vi "请求刷新.vi"(4 "Error Out":errorcluster caption="Error in") -> (0 "title with pic":cluster{"字符串 2":string, "二维图片":picture}[](array[cluster]), 1 "error out":errorcluster, 2 "stories":T1(array[cluster]), 3 "URL":string, 5 "top_stories":cluster{"字符串 2":string, "二维图片":picture}[](array[cluster]))   [LabVIEW 2012]
uses:
  <vilib>/addons/WireFlow/_WF_ProgressBar.llb/MessageTextType.ctl
  <vilib>/addons/WireFlow/_WF_ProgressBar.llb/ProgressBar_WireFlow.lvclass
panel:
  in  "delay (0 ms)":i32=1000
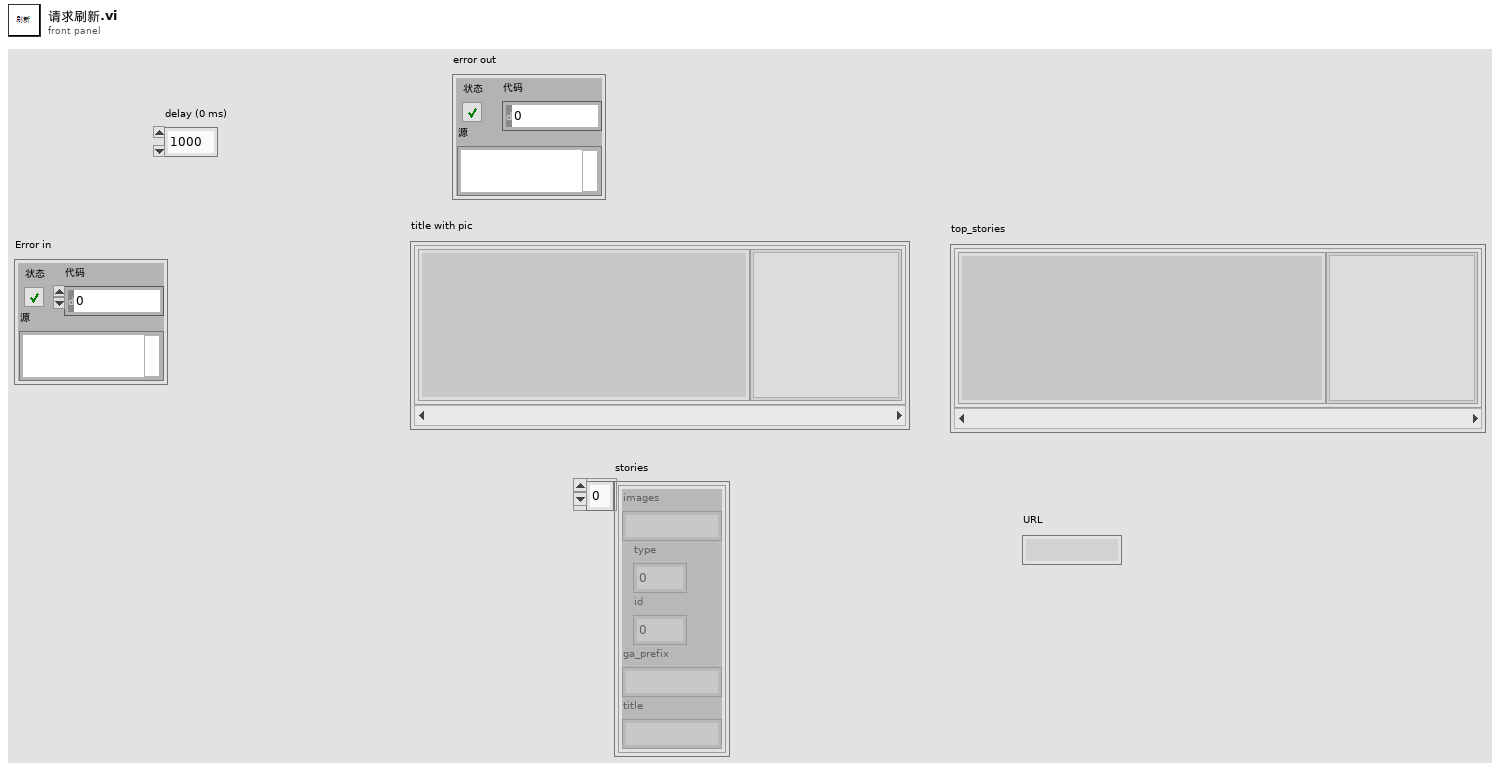
[diagram p1: front panel]
types:
  T1 = cluster{"images":string, "type":i32, "id":i64, "ga_prefix":string, "title":string}[]
  T2 = typedef "ProgressBar_WireFlow.lvclass/MessageTextType.ctl" = enum16{"Title", "General", "Current item"}
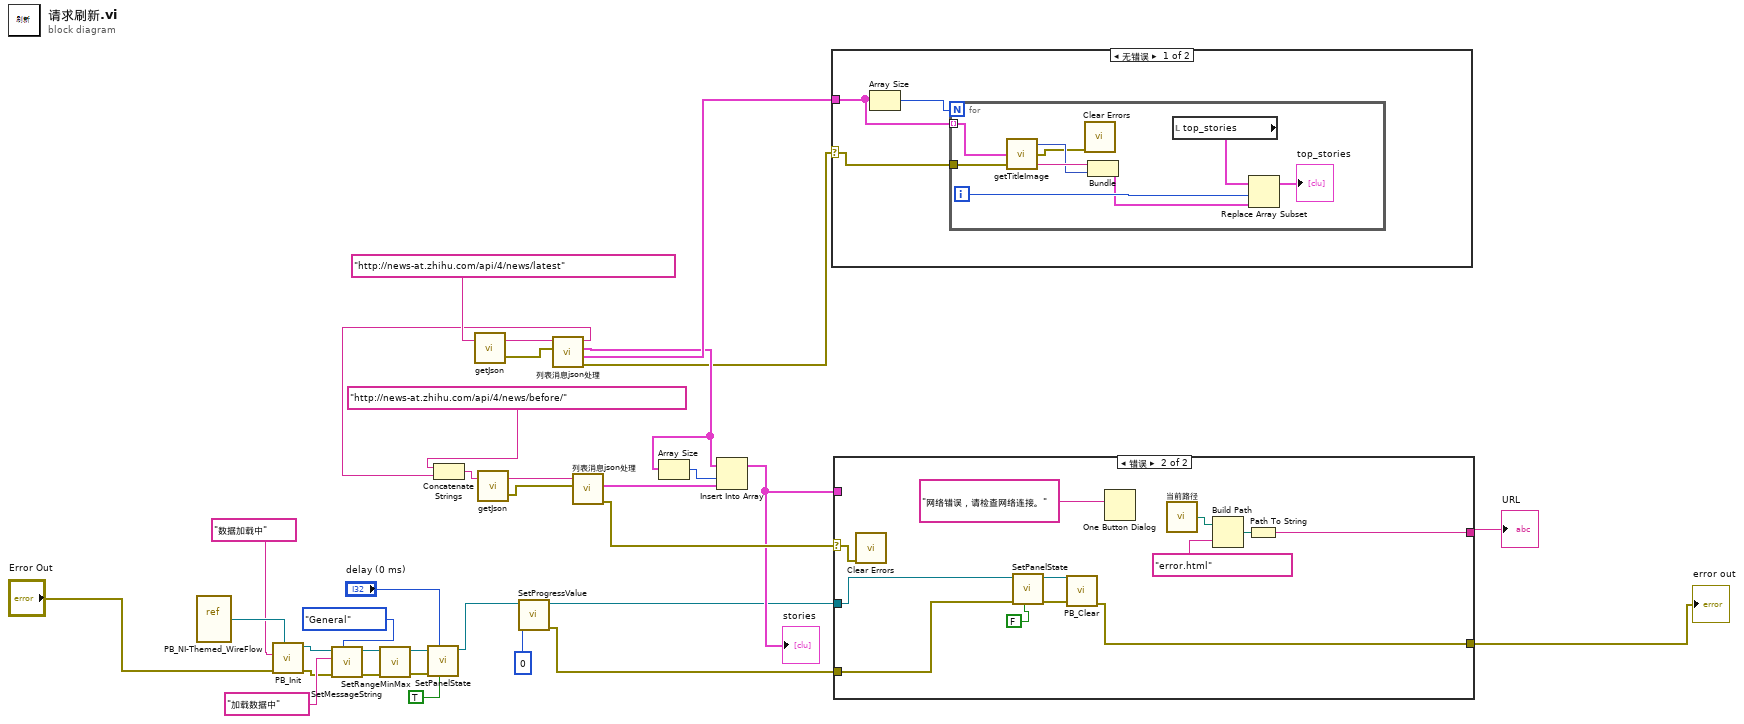
[diagram p0: block diagram]
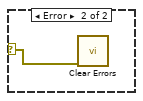
[diagram p2: hidden frame]
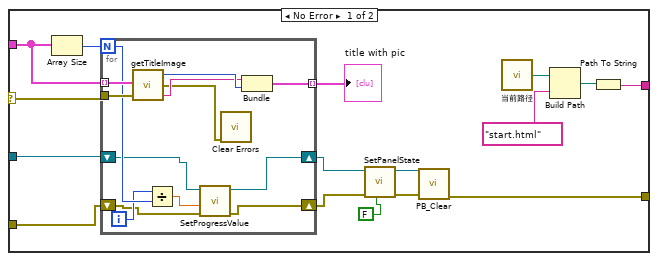
[diagram p3: hidden frame]
diagram:
  n1 = vi-ref "PB_NI-Themed_WireFlow.vi"() -> (w18:refnum<vi>)
  n2 = call <vilib>:"PB_Init.vi"("Progress VI"=w18, "error in (no error)"="Error Out", "title (\"Progress\")"="数据加载中") -> ("error out"=w11:errorcluster, "WF-ProgressBar out"=w16:refnum<class "ProgressBar_WireFlow.lvclass">)  [unwired: 7 in]
  n3 = call-dynamic "SetMessageString.vi"("message field"=MessageTextType."General", "error in (no error)"=w11, "Message"="加载数据中", "WF-ProgressBar in"=w16) -> ("error out"=w12:errorcluster, "WF-ProgressBar out"=w13:refnum<class "ProgressBar_WireFlow.lvclass">)  [unwired: 6 in]
  n4 = call-dynamic "SetRangeMinMax.vi"("error in (no error)"=w12, "WF-ProgressBar in"=w13) -> ("error out"=w9:errorcluster, "WF-ProgressBar out"=w10:refnum<class "ProgressBar_WireFlow.lvclass">)  [unwired: 8 in]
  n5 = call-dynamic "SetPanelState.vi"("State (T = Open)"=TRUE, "delay (0 ms)"="delay (0 ms)", "error in (no error)"=w9, "WF-ProgressBar in"=w10) -> ("WF-ProgressBar out"=w6:refnum<class "ProgressBar_WireFlow.lvclass">)  [unwired: 6 in, 1 out]
  n6 = call "getJson.vi"("URL"="http://news-at.zhihu.com/api/4/news/latest") -> ("error out"=w32:errorcluster, "响应体"=w33:string)  [unwired: 1 in]
  n7 = call-dynamic "SetProgressValue.vi"("Value"=0, "WF-ProgressBar in"=w6) -> ("error out"=w3:errorcluster, "WF-ProgressBar out"=w4:refnum<class "ProgressBar_WireFlow.lvclass">)  [unwired: 7 in, 1 out]
  n8 = call "列表消息json处理.vi"("error in (no error)"=w32, "json input"=w33) -> ("error out"=w22:errorcluster, "top_stories"=w31:T1, "stories"=w24:T1, "date"=w29:string)  [unwired: 2 in]
  n9 = Concatenate Strings("http://news-at.zhihu.com/api/4/news/before/", w29) -> (w30:string)
  n10 = call "getJson.vi"("URL"=w30) -> ("error out"=w26:errorcluster, "响应体"=w27:string)  [unwired: 1 in]
  n11 = call "列表消息json处理.vi"("error in (no error)"=w26, "json input"=w27) -> ("error out"=w23:errorcluster, "stories"=w21:T1)  [unwired: 2 in, 2 out]
  n12 = Array Size(array=w24) -> (size(s)=w25:i32)
  n13 = Insert Into Array(array=w24, index=w25, new element=w21) -> (w19:T1)
  "stories" <- w19
  n14 = case shown="无错误" w22 {
    selector: w22 -> [w35 w47]
    tunnel: w31 -> [w36 _]
    frame No Error {
      n15 = Array Size(array=w36) -> (size(s)=w37:i32)
      n16 = for {
        N: w37 -> [_]
        tunnel: w36 -> [w41] mode=indexing
        tunnel: w35 -> [w38]
        i -> [w45]
        n17 = call "getTitleImage.vi"("error in (no error)"=w38, "story"=w41) -> ("title"=w46:string, "error out"=w39:errorcluster, "图片"=w42:picture)  [unwired: 1 in]
        n18 = call <vilib>:"Clear Errors.vi"("error in (no error)"=w39) -> ()  [unwired: 6 in, 1 out]
        n19 = Bundle("title"=w46, "图片"=w42) -> (w44:cluster{"title":string, "图片":picture})  [unwired: 1 in]
        n20 = local read "top_stories"() -> (w43:cluster{"字符串 2":string, "二维图片":picture}[])
        n21 = Replace Array Subset(array=w43, new element=w44, index=w45) -> (→"top_stories":cluster{"字符串 2":string, "二维图片":picture}[])
      }
    }
    frame Error {
      n22 = call <vilib>:"Clear Errors.vi"("error in (no error)"=w47) -> ()  [unwired: 6 in, 1 out]
    }
  }
  n23 = case shown="错误" w23 {
    selector: w23 -> [w62 w88]
    tunnel: w19 -> [w61 _]
    tunnel: [w56 w83] -> w20
    tunnel: w4 -> [w55 w79]
    tunnel: w3 -> [w54 w78]
    tunnel: [w48 w77] -> w2
    frame No Error {
      n24 = Array Size(array=w61) -> (size(s)=w63:i32)
      n25 = for {
        N: w63 -> [w71]
        tunnel: w61 -> [w72] mode=indexing
        tunnel: w62 -> [w76]
        tunnel: [w73] -> w60 mode=indexing
        shift-right: [w68] -> w53
        shift-left: w55 -> [w67]
        shift-right: [w66] -> w52
        shift-left: w54 -> [w65]
        i -> [w70]
        n26 = call "getTitleImage.vi"("error in (no error)"=w76, "story"=w72) -> ("title"=w74:string, "error out"=w64:errorcluster, "图片"=w75:picture)  [unwired: 1 in]
        n27 = Divide(x=w70, y=w71) -> (x/y=w69:dbl)
        n28 = call-dynamic "SetProgressValue.vi"("error in (no error)"=w65, "Value"=w69, "WF-ProgressBar in"=w67) -> ("error out"=w66:errorcluster, "WF-ProgressBar out"=w68:refnum<class "ProgressBar_WireFlow.lvclass">)  [unwired: 6 in, 1 out]
        n29 = call <vilib>:"Clear Errors.vi"("error in (no error)"=w64) -> ()  [unwired: 6 in, 1 out]
        n30 = Bundle("title"=w74, "图片"=w75) -> (w73:cluster{"title":string, "图片":picture})  [unwired: 1 in]
      }
      "title with pic" <- w60
      n31 = call-dynamic "SetPanelState.vi"("State (T = Open)"=FALSE, "error in (no error)"=w52, "WF-ProgressBar in"=w53) -> ("error out"=w49:errorcluster, "WF-ProgressBar out"=w50:refnum<class "ProgressBar_WireFlow.lvclass">)  [unwired: 7 in]
      n32 = call-dynamic "PB_Clear.vi"("error in (no error)"=w49, "WF-ProgressBar in"=w50) -> ("error out"=w48:errorcluster)  [unwired: 8 in, 1 out]
      n33 = call "当前路径.vi"() -> ("路径"=w59:path)
      n34 = Build Path(base path=w59, name or relative path="start.html") -> (appended path=w57:path)
      n35 = Path To String(path=w57) -> (string=w56:string)
    }
    frame Error {
      n36 = call <vilib>:"Clear Errors.vi"("error in (no error)"=w88) -> ()  [unwired: 6 in, 1 out]
      n37 = call-dynamic "SetPanelState.vi"("State (T = Open)"=FALSE, "error in (no error)"=w78, "WF-ProgressBar in"=w79) -> ("error out"=w82:errorcluster, "WF-ProgressBar out"=w81:refnum<class "ProgressBar_WireFlow.lvclass">)  [unwired: 7 in]
      n38 = call-dynamic "PB_Clear.vi"("error in (no error)"=w82, "WF-ProgressBar in"=w81) -> ("error out"=w77:errorcluster)  [unwired: 8 in, 1 out]
      n39 = One Button Dialog(message="网络错误，请检查网络连接。") -> ()  [unwired: 1 in, 1 out]
      n40 = call "当前路径.vi"() -> ("路径"=w86:path)
      n41 = Build Path(base path=w86, name or relative path="error.html") -> (appended path=w84:path)
      n42 = Path To String(path=w84) -> (string=w83:string)
    }
  }
  "URL" <- w20
  "error out" <- w2
